vi "Send Block Length.vi"(8 "error in (no error)":errorcluster, 9 "Block Size In":u32, 10 "Array in":u8[][](array[numeric]), 11 "Refnum in":refnum<k21>) -> (0 "error out":errorcluster, 1 "Array Out":u8[][](array[numeric]) format="%.0x", 2 "Block Size Out":u32, 3 "Array out":string[](array[string]))   [LabVIEW 2014]
uses:
  <vilib>/xnet/xnet.llb/XNET Frame CAN.ctl
  <vilib>/xnet/xnet.llb/XNET Frame Type CAN.ctl
  <vilib>/xnet/xnet.llb/XNET Write (Frame CAN).vi
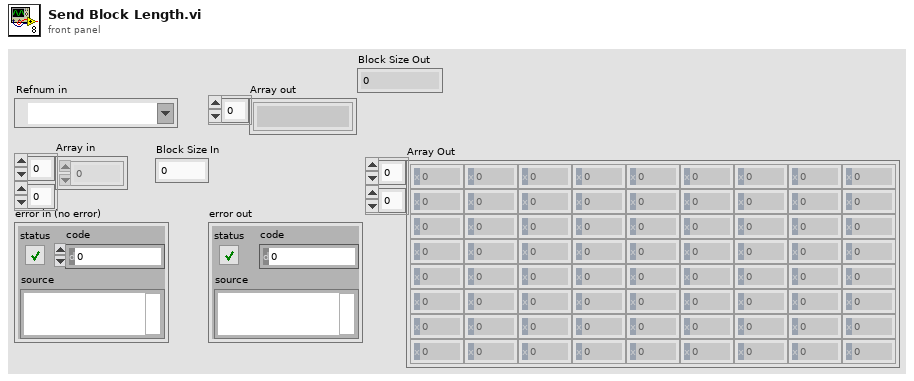
[diagram p1: front panel]
types:
  T1 = typedef "XNET Frame CAN.ctl" = cluster{"timestamp":timestamp, "payload":u8[], "identifier":u32, "type":T2, "extended?":bool, "echo?":bool}
  T2 = typedef "XNET Frame Type CAN.ctl" = u8
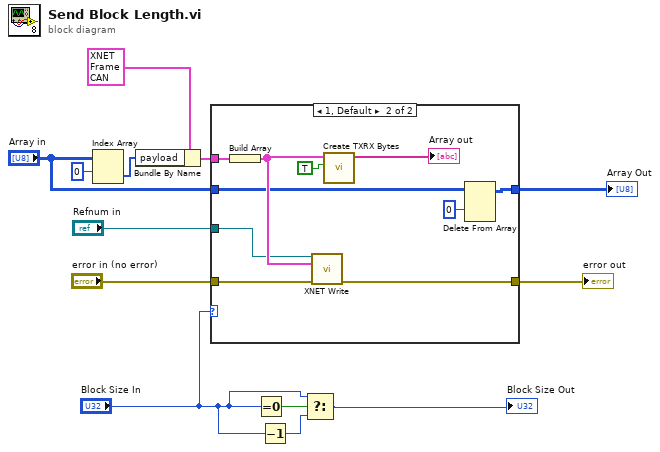
[diagram p0: block diagram]
diagram:
  n1 = Index Array(array="Array in", index (row)=0) -> (element=w7:u8[])  [unwired: 1 in]
  n2 = Bundle By Name(cluster=T1 {"timestamp"=timestamp(0 s since 1904-01-01), "payload"=[2, 39, 3, 85, 85, 85, 85, 85], "identifier"=402391172, "type"=0, "extended?"=TRUE, "echo?"=FALSE} ("Tx CAN frame"), "payload"=w7) -> (w10:T1)
  n3 = case shown="1, Default" "Block Size In" {
    tunnel: "error in (no error)" -> [w15 w25]
    tunnel: [w15 w24] -> w12
    tunnel: "Refnum in" -> [_ w20]
    tunnel: w10 -> [_ w19]
    tunnel: [w14 w17] -> w6
    tunnel: "Array in" -> [w14 w18]
    frame 0 {
    }
    frame 1, Default {
      n4 = Build Array(w19) -> (w22:T1[])
      n5 = call-poly <vilib>:"XNET Write.vi"("session in"=w20, "data"=w22, "error in (no error)"=w25) -> ("error out"=w24:errorcluster)  [unwired: 11 in, 1 out]
      n6 = call "Create TXRX Bytes.vi"("Cluster Array in"=w22, "Tx?"=TRUE) -> ("Array"=→"Array out":string[])  [unwired: 6 in, 2 out]
      n7 = Delete From Array(array=w18, index (row)=0) -> (array with subset deleted=w17:u8[][])  [unwired: 2 in, 1 out]
    }
  }
  "error out" <- w12
  "Array Out" <- w6
  n8 = Equal To 0?(x="Block Size In") -> (x = 0?=w5:bool)
  n9 = Decrement(x="Block Size In") -> (x-1=w3:u32)
  n10 = Select(t="Block Size In", s=w5, f=w3) -> (s? t:f=→"Block Size Out":u32)
